vi "428.vi"() -> ()   [LabVIEW 2015]
uses:
  0222 version 14/PF200/71421/Control 6.ctl
  0222 version 14/PF200/71421/Control 8.ctl
  0222 version 14/PF200/71421/Control 7.ctl
  0222 version 14/PF200/71421/Control 9.ctl
  0222 version 14/PF200/71421/Control 10.ctl
  0222 version 14/PF200/71421/Control 11.ctl
  0222 version 14/PF200/71421/Control 12.ctl
  <vilib>/addons/control/pid/pid.llb/PID (DBL).vi
  <vilib>/addons/control/pid/NI_PID_pid.lvlib
panel:
  out "Save File Path 2":path=path "C:/1.tdms"
  out "24 [NTU]":dbl
  out "23 [NTU]":dbl
  out "21 [NTU]":dbl
  in  "Ripen time [s]":dbl
  in  "Backwash time [s]":dbl
  out "Last backwash":timestamp
  in  "Filtered quality target [NTU]":dbl
  out "Coagulant [mg Al/L]":dbl(graph)
  in  "Coagulant PID gains":T1={"proportional gain (Kc)"=1.0, "integral time (Ti, min)"=0.01, "derivative time (Td, min)"=0.0} {"derivative time (Td, min)" format="%.3f"; "integral time (Ti, min)" format="%.3f"; "proportional gain (Kc)" format="%.3f"}
  out "Turbidities":dbl[][](graph)
  in  "Coagulant control":bool
  in  "Backwash control":bool
  out "UV 254":dbl[][](graph)
  in  "Sludge control":bool
  in  "Sludge flow [L/min]":dbl
  in  "Sludge PID gains":T1={"proportional gain (Kc)"=1.0, "integral time (Ti, min)"=0.01, "derivative time (Td, min)"=0.0} {"derivative time (Td, min)" format="%.3f"; "integral time (Ti, min)" format="%.3f"; "proportional gain (Kc)" format="%.3f"}
  in  "Main PID gains":T1={"proportional gain (Kc)"=1.0, "integral time (Ti, min)"=0.01, "derivative time (Td, min)"=0.0} {"derivative time (Td, min)" format="%.3f"; "integral time (Ti, min)" format="%.3f"; "proportional gain (Kc)" format="%.3f"}
  in  "Flow control":bool
  in  "Main flow [L/min]":dbl
  out "Main valve":dbl(graph)
  out "Filter head loss":dbl
  out "Water flow value":dbl
  out "Sludge flow value":dbl
  in  "Settled quality target [NTU]":dbl
  in  "Coagulant  [V]":dbl(slide) scale=0.0..5.0
  in  "Sludge valve [V]":dbl(slide) scale=0.0..5.0
  in  "Main valve [V]":dbl(slide) scale=0.0..5.0
  in  "backwash [ON/OFF]":bool
  out "Sludge valve":dbl(graph)
  out "Sludge flow meter":dbl[][](graph)
  out "Filter head loss":dbl[][](graph)
  out "Main flow meter":dbl[][](graph)
  out "error out":errorcluster
  in  "Stop Experiment":bool
  in  "Input: Seconds per data point (sec)":dbl
  in  "Start Experiment":bool
  in  "Exit":bool
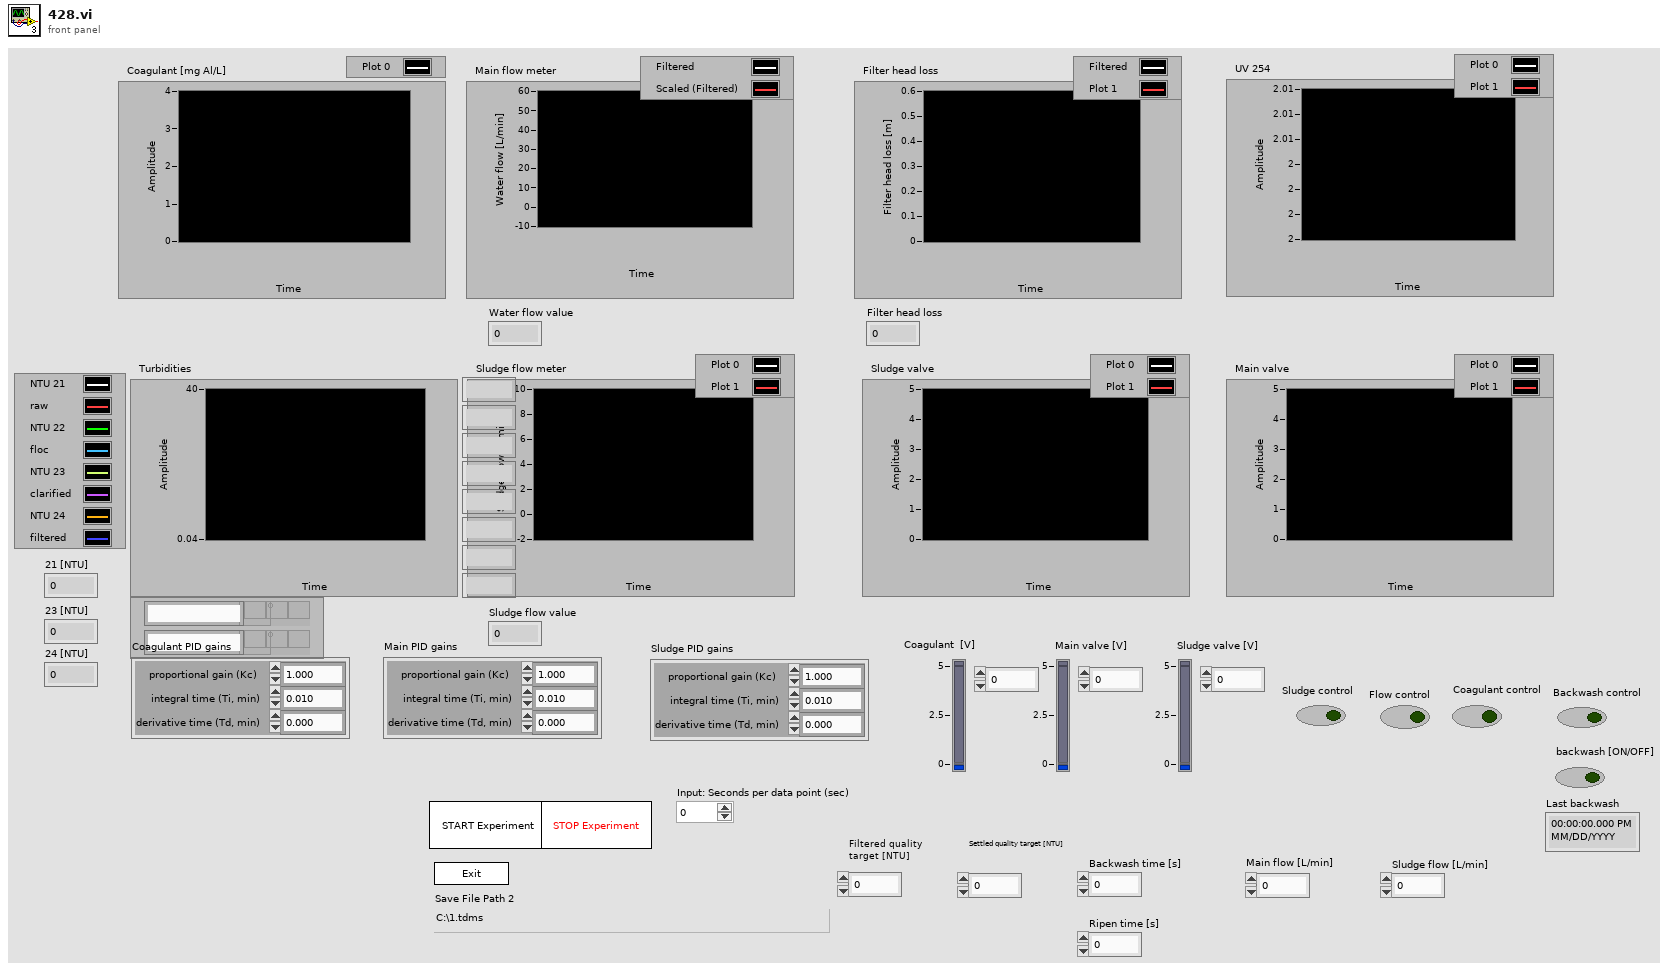
[diagram p1: front panel]
types:
  T1 = cluster{"proportional gain (Kc)":dbl, "integral time (Ti, min)":dbl, "derivative time (Td, min)":dbl}
  T2 = typedef "Control 8.ctl" = cluster{"Boolean <Replace Me>":bool, "String <Replace Me>":string, "Numeric <Replace Me>":dbl}
  T3 = typedef "Control 6.ctl" = enum16{"Initialize", "Wait for Event", "Experiment", "Exit"}
  T4 = typedef "Control 7.ctl" = enum16{"Initialize", "Wait for Event", "Experiment", "Exit"}
  T5 = typedef "Control 9.ctl" = enum16{"Initialize", "Wait for Event", "Experiment", "Exit"}
  T6 = typedef "Control 10.ctl" = enum16{"Initialize", "Wait for Event", "Experiment", "Exit"}
  T7 = enum16{"open", "open or create", "create or replace", "create", "open (read-only)"}
  T8 = typedef "Control 11.ctl" = enum16{"Initialize", "Wait for Event", "Experiment", "Exit"}
  T9 = typedef "Control 12.ctl" = enum16{"Initialize", "Wait for Event", "Experiment", "Exit"}
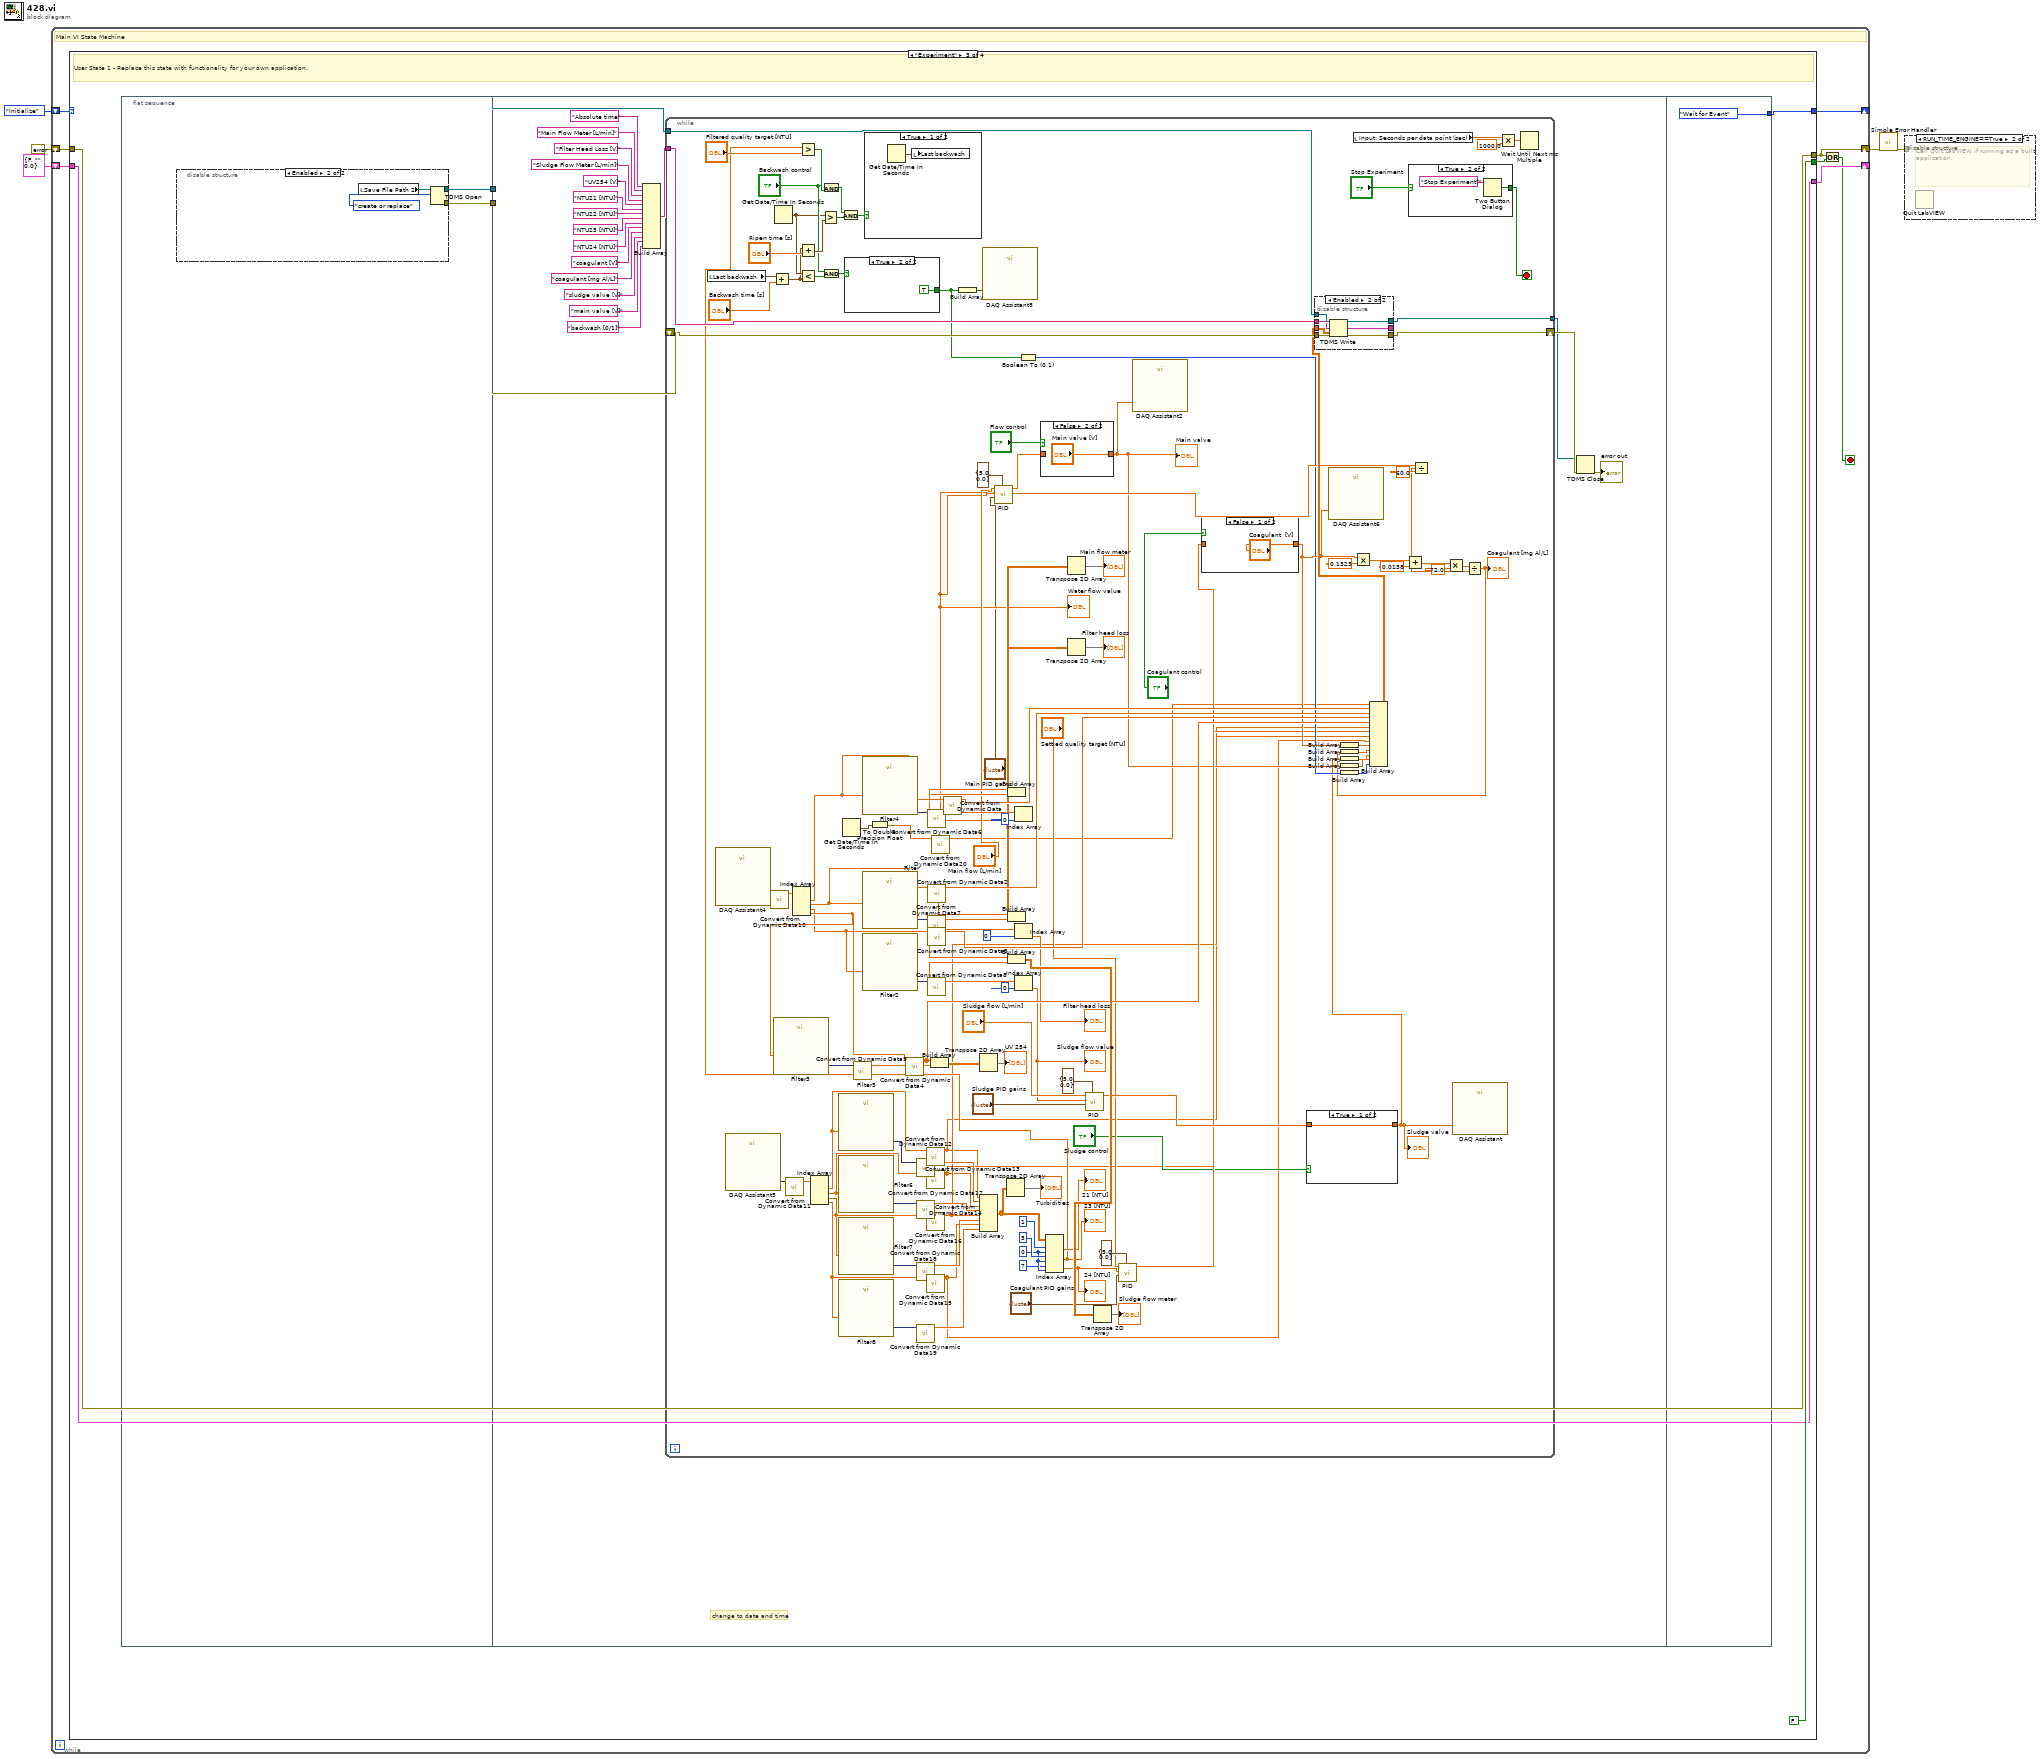
[diagram p0: block diagram]
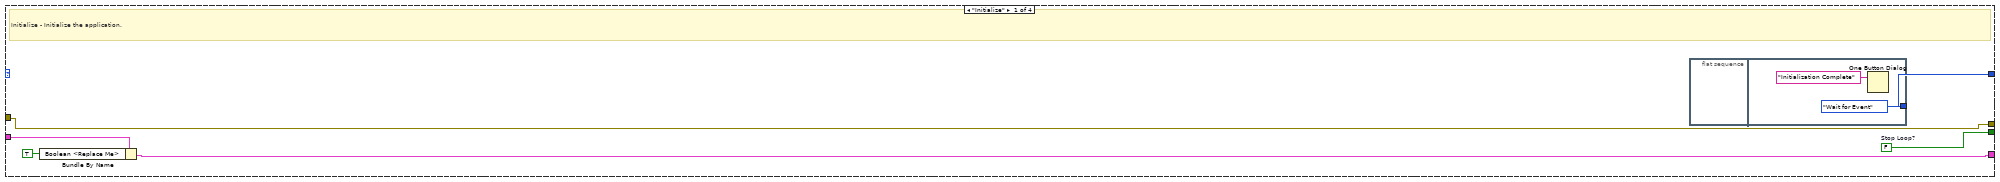
[diagram p3: hidden frame]
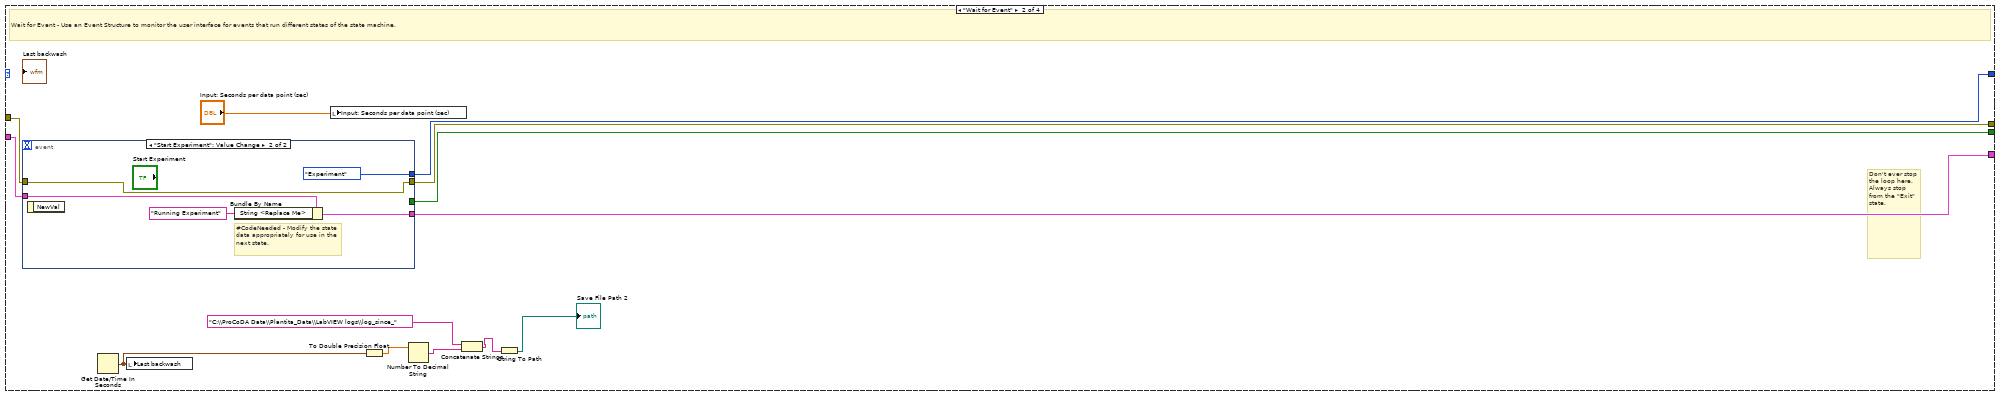
[diagram p4: hidden frame]
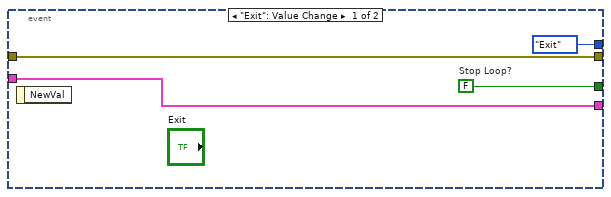
[diagram p5: hidden frame]
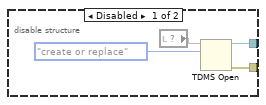
[diagram p6: hidden frame]
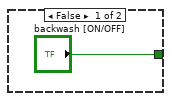
[diagram p7: hidden frame]
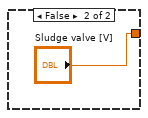
[diagram p10: hidden frame]
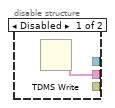
[diagram p12: hidden frame]
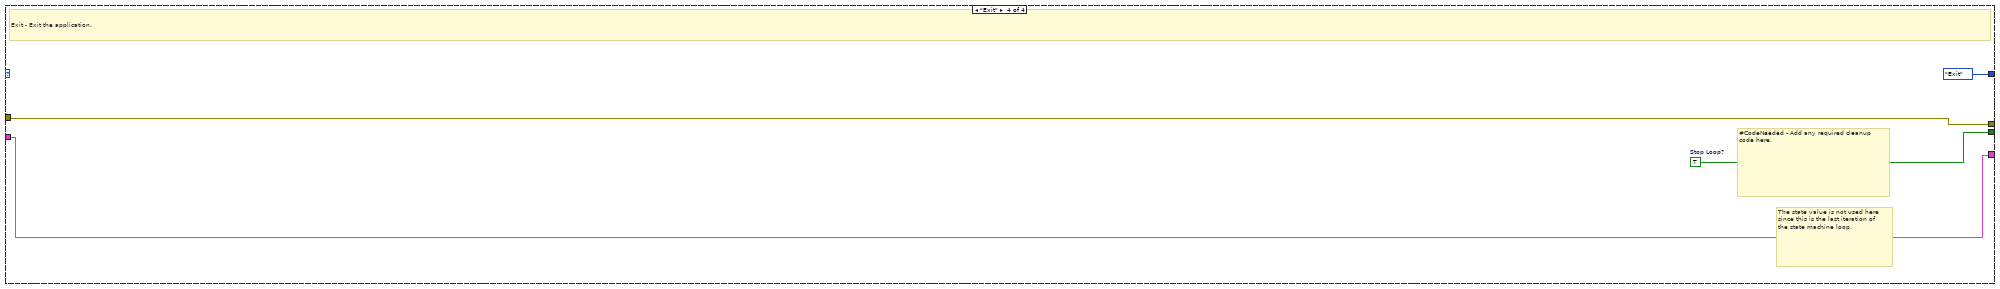
[diagram p14: hidden frame]
diagram:
  n1 = while {
    shift-right: [w12] -> _
    shift-left: Control_6."Initialize" ("Initial State") -> [w13]
    shift-right: [w10] -> _
    shift-left: T2 {"Boolean <Replace Me>"=FALSE, "String <Replace Me>"="", "Numeric <Replace Me>"=0.0} -> [w11]
    shift-right: [w6] -> w3
    shift-left: errorcluster {"status"=FALSE, "code"=0, "source"=""} ("error constant") -> [w9]
    stop <- w7 stop-if-true
    # "Main VI State Machine"
    n2 = case shown="\"Experiment\"" w13 {
      tunnel: [w14 w34 w46 Control_12."Exit" ("(Value Not Used)")] -> w12
      tunnel: [w19 w29 FALSE ("Stop Loop?") w229] -> w8
      tunnel: w11 -> [w18 w33 w48 w230]
      tunnel: [w17 w32 w48 w230] -> w10
      tunnel: w9 -> [w15 w31 w47 w228]
      tunnel: [w15 w30 w47 w228] -> w6
      frame "Initialize" {
        w19 = FALSE  # Stop Loop?
        # "Initialize - Initialize the application."
        n3 = Bundle By Name(cluster=w18, "Boolean <Replace Me>"=TRUE ("Replace_Me_Boolean")) -> (w17:T2)
        n4 = flat-sequence {
          tunnel: [Control_7."Wait for Event" ("Next State")] -> w14
          frame #0 {
          }
          frame #1 {
            n5 = One Button Dialog(message="Initialization Complete") -> ()  [unwired: 1 in, 1 out]
          }
        }
      }
      frame "Wait for Event" {
        # "Don't ever stop the loop here. Always stop from the \"Exit\" state."
        # "Wait for Event - Use an Event Structure to monitor the user interface for events that run different states of the state machine."
        n6 = event shown="[1] \"Start Experiment\": Value Change" {
          selector: _ -> [_ _]
          dyn-events: _ -> [_ _]
          timeout: _ -> [_ _]
          tunnel: [Control_9."Exit" ("Next State") Control_10."Experiment" ("Next State")] -> w34
          tunnel: w33 -> [w37 w42]
          tunnel: [w37 w41] -> w32
          tunnel: w31 -> [w36 w39]
          tunnel: [w36 w39] -> w30
          tunnel: [w35 _] -> w29
          event "Exit": Value Change {
            w35 = FALSE  # Stop Loop?
            n7 = event-data() -> ()  [unwired: 1 in, 1 out]
          }
          event "Start Experiment": Value Change {
            # "#CodeNeeded - Modify the state data appropriately for use in the next state."
            n8 = event-data() -> ()  [unwired: 1 in, 1 out]
            n9 = Bundle By Name(cluster=w42, "String <Replace Me>"="Running Experiment" ("Running User State 1")) -> (w41:T2)
          }
        }
        n10 = Get Date/Time In Seconds() -> (seconds since 1Jan1904=w27:timestamp)
        n11 = local write "Last backwash"(w27) -> ()
        n12 = local write "Input: Seconds per data point (sec)"("Input: Seconds per data point (sec)") -> ()
        n13 = To Double Precision Float(number=w27) -> (double precision float=w25:dbl)
        n14 = Number To Decimal String(number=w25) -> (decimal integer string=w24:string)  [unwired: 1 in]
        n15 = Concatenate Strings("C:\\ProCoDA Data\\Plantita_Data\\LabVIEW logs\\log_since_", w24) -> (w23:string)
        n16 = String To Path(string=w23) -> (path=→"Save File Path 2":path)
      }
      frame "Experiment" {
        # "User State 1 - Replace this state with functionality for your own application."
        n17 = flat-sequence {
          tunnel: [w51] -> w45
          tunnel: [w50] -> w44
          tunnel: w45 -> [w77]
          tunnel: w44 -> [w79]
          tunnel: [Control_11."Wait for Event" ("Next State")] -> w46
          frame #0 {
            n18 = disable-structure shown="Enabled" {
              disable-tunnel: [w55 w57] -> w51
              disable-tunnel: [w54 w56] -> w50
              frame Disabled {
                n19 = local read item#-1() -> (w53)
                n20 = TDMS Open(10:T7."create or replace" ("operation (0:open)"), 11:w53) -> (0:w54:errorcluster, 3:w55:refnum<k34>)  [unwired: 5 in]
              }
              frame Enabled {
                n21 = local read "Save File Path 2"() -> (w59:path)
                n22 = TDMS Open(10:T7."create or replace" ("operation (0:open)"), 11:w59) -> (0:w56:errorcluster, 3:w57:refnum<k34>)  [unwired: 5 in]
              }
            }
          }
          frame #1 {
            # "change to date and time"
            n23 = Build Array("Absolute time", "Main Flow Meter [L/min]", "Filter Head Loss [V]", "Sludge Flow Meter [L/min]", "UV254 [V]" ("element"), "NTU21 [NTU]", "NTU22 [NTU]", "NTU23 [NTU]", "NTU24 [NTU]" ("element"), "coagulant [V]" ("element"), "coagulant [mg Al/L]" ("element"), "sludge valve [V]" ("element"), "main valve [V]" ("element"), "backwash [0/1]" ("element")) -> (w78:string[])
            n24 = while {
              shift-right: [w194] -> w75
              shift-left: w79 -> [w197]
              tunnel: w78 -> [w195]
              tunnel: w77 -> [w196]
              tunnel: [w193] -> w74
              stop <- w198 stop-if-true
              w103 = 0 ("disabled index (col)")
              n25 = local read "Last backwash"() -> (w118:timestamp)
              n26 = call "DAQ Assistant4"() -> ("data"=w166:dynamicdata)  [unwired: 17 in, 2 out]
              n27 = call "DAQ Assistant5"() -> ("data"=w153:dynamicdata)  [unwired: 17 in, 2 out]
              n28 = call "Convert from Dynamic Data10"("Dynamic Data Type"=w166) -> ("Array"=w167:dbl[])  [unwired: 3 in]
              n29 = Add(x=w118, y="Backwash time [s]") -> (x+y=w108:timestamp)
              n30 = Get Date/Time In Seconds() -> (seconds since 1Jan1904=w109:timestamp)
              n31 = call "Convert from Dynamic Data11"("Dynamic Data Type"=w153) -> ("Array"=w152:dbl[])  [unwired: 3 in]
              n32 = Index Array(array=w167) -> (element #1=w165:dbl, element #2=w157:dbl, element #3=w164:dbl, element #4=w168:dbl)  [unwired: 4 in]
              n33 = call "Filter3"("Signal"=w168) -> ("Filtered Signal"=w182:dynamicdata)  [unwired: 9 in, 1 out]
              n34 = Add(x=w108, y="Ripen time [s]") -> (x+y=w116:timestamp)
              n35 = Less?(x=w109, y=w108) -> (x < y?=w110:bool)
              n36 = Index Array(array=w152) -> (element #1=w151:dbl, element #2=w146:dbl, element #3=w143:dbl, element #4=w137:dbl)  [unwired: 4 in]
              n37 = Greater?(x=w109, y=w116) -> (0:w114:bool)
              n38 = And(x="Backwash control", y=w110) -> (x .and. y?=w107:bool)
              n39 = call "Filter5"("Signal"=w151) -> ("Filtered Signal"=w150:dynamicdata)  [unwired: 9 in, 1 out]
              n40 = call "Filter6"("Signal"=w146) -> ("Filtered Signal"=w145:dynamicdata)  [unwired: 9 in, 1 out]
              n41 = call "Filter7"("Signal"=w143) -> ("Filtered Signal"=w140:dynamicdata)  [unwired: 9 in, 1 out]
              n42 = call "Filter8"("Signal"=w137) -> ("Filtered Signal"=w138:dynamicdata)  [unwired: 9 in, 1 out]
              n43 = Get Date/Time In Seconds() -> (seconds since 1Jan1904=w142:timestamp)
              n44 = case shown="True" w107 {
                tunnel: ["backwash [ON/OFF]" TRUE ("backwash [ON/OFF]")] -> w92
                frame False {
                }
                frame True {
                }
              }
              n45 = call "Convert from Dynamic Data9"("Dynamic Data Type"=w182) -> ("Array"=w177:dbl[])  [unwired: 3 in]
              n46 = call "Filter4"("Signal"=w165) -> ("Filtered Signal"=w191:dynamicdata)  [unwired: 9 in, 1 out]
              n47 = call "Filter"("Signal"=w157) -> ("Filtered Signal"=w186:dynamicdata)  [unwired: 9 in, 1 out]
              n48 = call "Filter2"("Signal"=w164) -> ("Filtered Signal"=w183:dynamicdata)  [unwired: 9 in, 1 out]
              n49 = To Double Precision Float(number=w142) -> (double precision float=w141:dbl)
              n50 = call "Convert from Dynamic Data4"("Dynamic Data Type"=w168) -> ("Array"=w178:dbl[])  [unwired: 3 in]
              n51 = call "Convert from Dynamic Data13"("Dynamic Data Type"=w150) -> ("Array"=w147:dbl[])  [unwired: 3 in]
              n52 = call "Convert from Dynamic Data14"("Dynamic Data Type"=w145) -> ("Array"=w144:dbl[])  [unwired: 3 in]
              n53 = call "Convert from Dynamic Data18"("Dynamic Data Type"=w140) -> ("Array"=w139:dbl[])  [unwired: 3 in]
              n54 = call "Convert from Dynamic Data19"("Dynamic Data Type"=w138) -> ("Array"=w136:dbl[])  [unwired: 3 in]
              n55 = call "Convert from Dynamic Data12"("Dynamic Data Type"=w151) -> ("Array"=w80:dbl[])  [unwired: 3 in]
              n56 = call "Convert from Dynamic Data17"("Dynamic Data Type"=w146) -> ("Array"=w81:dbl[])  [unwired: 3 in]
              n57 = call "Convert from Dynamic Data16"("Dynamic Data Type"=w143) -> ("Array"=w82:dbl[])  [unwired: 3 in]
              n58 = call "Convert from Dynamic Data15"("Dynamic Data Type"=w137) -> ("Array"=w83:dbl[])  [unwired: 3 in]
              n59 = call "Convert from Dynamic Data6"("Dynamic Data Type"=w191) -> ("Array"=w175:dbl[])  [unwired: 3 in]
              n60 = call "Convert from Dynamic Data7"("Dynamic Data Type"=w186) -> ("Array"=w170:dbl[])  [unwired: 3 in]
              n61 = call "Convert from Dynamic Data8"("Dynamic Data Type"=w183) -> ("Array"=w169:dbl[])  [unwired: 3 in]
              n62 = call "Convert from Dynamic Data2"("Dynamic Data Type"=w157) -> ("Array"=w187:dbl[])  [unwired: 3 in]
              n63 = call "Convert from Dynamic Data3"("Dynamic Data Type"=w164) -> ("Array"=w181:dbl[])  [unwired: 3 in]
              n64 = Build Array(w178, w177) -> (w176:dbl[][])
              n65 = call "Convert from Dynamic Data20"("Dynamic Data Type"=w141) -> ("Array"=w89:dbl[])  [unwired: 3 in]
              n66 = call "Convert from Dynamic Data"("Dynamic Data Type"=w165) -> ("Array"=w188:dbl[])  [unwired: 3 in]
              n67 = Build Array(w92) -> (w96:bool[])
              n68 = Transpose 2D Array(2D array=w176) -> (transposed array=→"UV 254":dbl[][])
              n69 = Build Array(w80, w147, w81, w144, w82, w139, w83, w136) -> (w106:dbl[][])
              n70 = call "DAQ Assistant8"("data"=w96) -> ()  [unwired: 17 in, 2 out]
              n71 = Transpose 2D Array(2D array=w106) -> (transposed array=→"Turbidities":dbl[][])
              n72 = Build Array(w188, w175) -> (w189:dbl[][])
              n73 = Build Array(w187, w170) -> (w184:dbl[][])
              n74 = Build Array(w181, w169) -> (w180:dbl[][])
              n75 = Index Array(array=w175, index=0) -> (element=w126:dbl)
              "Water flow value" <- w126
              n76 = call-poly <vilib>:"PID.vi"("output range"=cluster{"output high":dbl, "output low":dbl} {"output high"=5.0, "output low"=0.0}, "PID gains"="Main PID gains", "process variable"=w126, "setpoint"="Main flow [L/min]") -> ("output"=w159:dbl)  [unwired: 6 in, 1 out]
              n77 = Index Array(array=w170, index=0) -> (element=→"Filter head loss":dbl)
              n78 = Index Array(array=w169, index=0) -> (element=w149:dbl)
              "Sludge flow value" <- w149
              n79 = Boolean To (0,1)(Boolean=w92) -> (0, 1=w93:i16)
              n80 = case shown="False" "Flow control" {
                tunnel: [w209 "Main valve [V]"] -> w94
                tunnel: w159 -> [w209 _]
                frame True {
                }
                frame False {
                }
              }
              "Main valve" <- w94
              n81 = Index Array(array=w106, index (row) #1=1 ("index (row)"), index (col) #1=w103, index (row) #2=5 ("disabled index (row)"), index (col) #2=w103, index (row) #3=7 ("disabled index (row)"), index (col) #3=w103) -> (element #1=→"21 [NTU]":dbl, element #2=w97:dbl, element #3=w99:dbl)
              "23 [NTU]" <- w97
              "24 [NTU]" <- w99
              n82 = Greater?(x=w97, y="Filtered quality target [NTU]") -> (0:w120:bool)
              n83 = And(x="Backwash control", y=w120) -> (x .and. y?=w112:bool)
              n84 = And(x=w112, y=w114) -> (x .and. y?=w113:bool)
              n85 = case shown="True" w113 {
                frame True {
                  n86 = Get Date/Time In Seconds() -> (seconds since 1Jan1904=w204:timestamp)
                  n87 = local write "Last backwash"(w204) -> ()
                }
                frame False {
                }
              }
              n88 = Transpose 2D Array(2D array=w189) -> (transposed array=→"Main flow meter":dbl[][])
              n89 = Transpose 2D Array(2D array=w184) -> (transposed array=→"Filter head loss":dbl[][])
              n90 = call-poly <vilib>:"PID.vi"("output range"=cluster{"output high":dbl, "output low":dbl} {"output high"=5.0, "output low"=0.0}, "PID gains"="Sludge PID gains", "process variable"=w149, "setpoint"="Sludge flow [L/min]") -> ("output"=w158:dbl)  [unwired: 6 in, 1 out]
              n91 = Transpose 2D Array(2D array=w180) -> (transposed array=→"Sludge flow meter":dbl[][])
              n92 = call-poly <vilib>:"PID.vi"("output range"=cluster{"output high":dbl, "output low":dbl} {"output high"=5.0, "output low"=0.0}, "PID gains"="Coagulant PID gains", "process variable"=w99, "setpoint"="Settled quality target [NTU]") -> ("output"=w132:dbl)  [unwired: 6 in, 1 out]
              n93 = call "DAQ Assistant2"("data"=w94) -> ()  [unwired: 17 in, 2 out]
              n94 = case shown="False" "Coagulant control" {
                tunnel: w132 -> [_ w206]
                tunnel: ["Coagulant  [V]" w206] -> w95
                frame False {
                }
                frame True {
                }
              }
              n95 = case shown="True" "Sludge control" {
                tunnel: [w207 "Sludge valve [V]"] -> w91
                tunnel: w158 -> [w207 _]
                frame True {
                }
                frame False {
                }
              }
              "Sludge valve" <- w91
              n96 = call "DAQ Assistant6"("data"=w95) -> ()  [unwired: 17 in, 2 out]
              n97 = Build Array(w95) -> (w84:dbl[])
              n98 = Build Array(w91) -> (w86:dbl[])
              n99 = Build Array(w94) -> (w87:dbl[])
              n100 = Build Array(w93) -> (w88:i16[])
              n101 = local read "Input: Seconds per data point (sec)"() -> (w199:dbl)
              n102 = Multiply(x=w95, y=0.1323) -> (x*y=w129:dbl)
              n103 = Add(x=w129, y=0.0138) -> (x+y=w124:dbl)
              n104 = case shown="True" "Stop Experiment" {
                selector: "Stop Experiment" -> [w224 _]
                tunnel: [w224 w226] -> w198
                frame False {
                }
                frame True {
                  n105 = Two Button Dialog(message="Stop Experiment?") -> (T button?=w226:bool)  [unwired: 2 in]
                }
              }
              n106 = Divide(x=w126, y=60.0) -> (x/y=w125:dbl)
              n107 = Multiply(x=w124, y=72.0) -> (x*y=w123:dbl)
              n108 = call "DAQ Assistant"("data"=w91) -> ()  [unwired: 17 in, 2 out]
              n109 = Divide(x=w123, y=w125) -> (x/y=w90:dbl)
              "Coagulant [mg Al/L]" <- w90
              n110 = Build Array(w90) -> (w85:dbl[])
              n111 = Build Array(w89, w188, w187, w181, w178, w80, w81, w82, w83, w84, w85, w86, w87, w88) -> (w192:dbl[][])
              n112 = disable-structure shown="Enabled" {
                disable-tunnel: [w212 w219] -> _
                disable-tunnel: w197 -> [_ w223]
                disable-tunnel: [_ w222] -> w194
                disable-tunnel: [_ w221] -> w193
                disable-tunnel: w196 -> [_ w220]
                disable-tunnel: w195 -> [_ w218]
                disable-tunnel: w192 -> [_ w217]
                frame Disabled {
                  n113 = TDMS Write(7:w212) -> (0:w215:refnum<k34>, 4:w216:refnum<k34>, 9:w211:waveform(dbl)[], 11:w214:errorcluster, 15:w213:errorcluster)  [unwired: 2 in, 2 out]
                }
                frame Enabled {
                  n114 = TDMS Write(0:w220, 7:w218, 9:w217, 11:w223) -> (4:w221:refnum<k34>, 8:w219:string[], 15:w222:errorcluster)  [unwired: 2 in, 1 out]
                }
              }
              n115 = Multiply(x=w199, y=1000.0) -> (x*y=w201:dbl)
              n116 = Wait Until Next ms Multiple(millisecond multiple=w201) -> ()  [unwired: 1 out]
            }
            n117 = TDMS Close(8:w75, 11:w74) -> (0:→"error out":errorcluster)  [unwired: 1 out]
          }
          frame #2 {
          }
        }
      }
      frame "Exit" {
        w229 = TRUE  # Stop Loop?
        # "#CodeNeeded - Add any required cleanup code here."
        # "The state value is not used here since this is the last iteration of the state machine loop."
        # "Exit - Exit the application."
      }
    }
    n118 = Or(x=w6, y=w8) -> (x .or. y?=w7:bool)
  }
  n119 = call <vilib>:"Simple Error Handler.vi"("error in (no error)"=w3) -> ("error out"=w2:errorcluster)  [unwired: 4 in, 4 out]
  n120 = disable-structure shown="RUN_TIME_ENGINE==True" {
    disable-tunnel: w2 -> [_ _]
    frame condition #0 (active) {
    }
    frame condition #1 {
      # "Call Quit LabVIEW if running as a built application."
      n121 = Quit LabVIEW() -> ()  [unwired: 1 in]
    }
  }
